vi "Motor Accion.vi"(11 "Tipo Movimiento":string) -> ()   [LabVIEW 2013, in "Proyecto 2 Touch.lvrbt"]
uses:
  Proyecto 2 Touch.lvrbt
  <vilib>/NXT/LegoClasses/BrickReference/BrickReference.lvclass
  <vilib>/NXT/Subs/LVHSConnector.ctl
  <vilib>/NXT/NXTIO Xnodes/NXTIOXNode/NXTIO.xnode
  <vilib>/NXT/NXTIO Xnodes/AddressXNode/NXTIOAddress.xnode
  <vilib>/NXT/Block Support/NXT_OutputPort.ctl
  <vilib>/NXT/NXTIO Xnodes/NXTIONodeSubVIs/NXTMoveMotors.vi
  <vilib>/NXT/NXTIO Xnodes/NXTIONodeSubVIs/LEGOResetMotors.vi
  <vilib>/NXT/NXTIO Xnodes/NXTIONodeSubVIs/LEGOStopAllMotors.vi
  <vilib>/NXT/Dual Mode Library/Waits/Wait_Rotation.vi
  <vilib>/NXT/Dual Mode Library/Waits/Wait_Num(msec).vi
  Global Var.vi
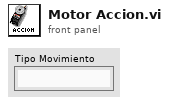
[diagram p1: front panel]
types:
  T1 = typedef "NXT_OutputPort.ctl" = u8
  T2 = typedef "LVHSConnector.ctl" = refnum<class "BrickReference.lvclass">
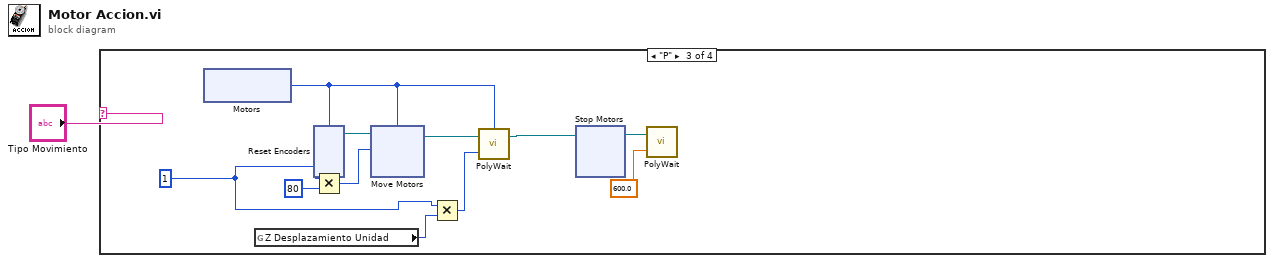
[diagram p0: block diagram]
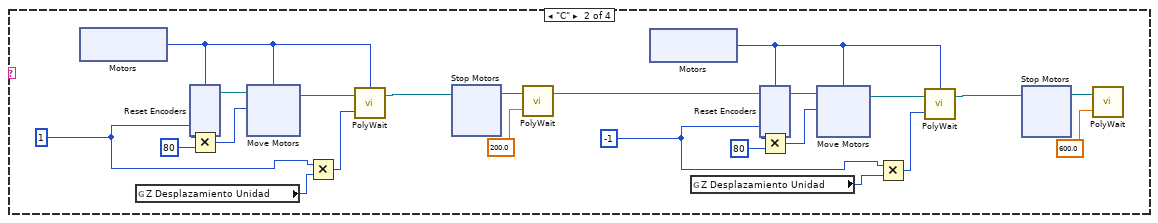
[diagram p3: hidden frame]
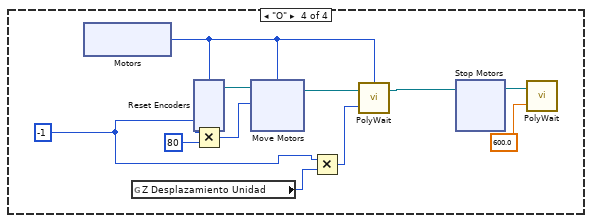
[diagram p4: hidden frame]
diagram:
  n1 = case shown="\"P\"" "Tipo Movimiento" {
    frame Default {
    }
    frame "C" {
      w7 = -1 ("x")
      w17 = 1 ("x")
      n2 = xnode "Motors"() -> ("Motor"=w16:T1)
      n3 = global read "Global Var.vi" "Z Desplazamiento Unidad"() -> (w2:i32)
      n4 = xnode "Reset Encoders"("Motors"=w16) -> ("NXT/EV3"=w23:T2)  [unwired: 1 in]
      n5 = Multiply(x=w17, y=80) -> (x*y=w19:i32)
      n6 = xnode "Move Motors"("Power/Speed 1"=w19, "Motors"=w16, "NXT/EV3"=w23) -> ("NXT/EV3"=w20:T2)
      n7 = Multiply(x=w17, y=w2) -> (x*y=w18:i32)
      n8 = call-poly <vilib>:"PolyWait.vi"("Position Change (180)"=w18, "NXT/EV3"=w20, "Port (Port A)"=w16) -> ("NXT/EV3"=w15:T2)  [unwired: 1 in]
      n9 = xnode "Stop Motors"("NXT/EV3"=w15) -> ("NXT/EV3"=w22:T2)  [unwired: 1 in]
      n10 = call-poly <vilib>:"PolyWait.vi"("Time (100 msec)"=sgl 200.0 ("Time (1 sec)"), "NXT/EV3"=w22) -> ("NXT/EV3"=w4:T2)  [unwired: 2 in]
      n11 = xnode "Motors"() -> ("Motor"=w6:T1)
      n12 = global read "Global Var.vi" "Z Desplazamiento Unidad"() -> (w3:i32)
      n13 = xnode "Reset Encoders"("Motors"=w6, "NXT/EV3"=w4) -> ("NXT/EV3"=w13:T2)
      n14 = Multiply(x=w7, y=80) -> (x*y=w9:i32)
      n15 = xnode "Move Motors"("Power/Speed 1"=w9, "Motors"=w6, "NXT/EV3"=w13) -> ("NXT/EV3"=w10:T2)
      n16 = Multiply(x=w7, y=w3) -> (x*y=w8:i32)
      n17 = call-poly <vilib>:"PolyWait.vi"("Position Change (180)"=w8, "NXT/EV3"=w10, "Port (Port A)"=w6) -> ("NXT/EV3"=w5:T2)  [unwired: 1 in]
      n18 = xnode "Stop Motors"("NXT/EV3"=w5) -> ("NXT/EV3"=w12:T2)  [unwired: 1 in]
      n19 = call-poly <vilib>:"PolyWait.vi"("Time (100 msec)"=sgl 600.0 ("Time (1 sec)"), "NXT/EV3"=w12) -> ()  [unwired: 2 in, 1 out]
    }
    frame "P" {
      w58 = 1 ("x")
      n20 = xnode "Motors"() -> ("Motor"=w57:T1)
      n21 = global read "Global Var.vi" "Z Desplazamiento Unidad"() -> (w55:i32)
      n22 = xnode "Reset Encoders"("Motors"=w57) -> ("NXT/EV3"=w64:T2)  [unwired: 1 in]
      n23 = Multiply(x=w58, y=80) -> (x*y=w60:i32)
      n24 = xnode "Move Motors"("Power/Speed 1"=w60, "Motors"=w57, "NXT/EV3"=w64) -> ("NXT/EV3"=w61:T2)
      n25 = Multiply(x=w58, y=w55) -> (x*y=w59:i32)
      n26 = call-poly <vilib>:"PolyWait.vi"("Position Change (180)"=w59, "NXT/EV3"=w61, "Port (Port A)"=w57) -> ("NXT/EV3"=w56:T2)  [unwired: 1 in]
      n27 = xnode "Stop Motors"("NXT/EV3"=w56) -> ("NXT/EV3"=w63:T2)  [unwired: 1 in]
      n28 = call-poly <vilib>:"PolyWait.vi"("Time (100 msec)"=sgl 600.0 ("Time (1 sec)"), "NXT/EV3"=w63) -> ()  [unwired: 2 in, 1 out]
    }
    frame "O" {
      w84 = -1 ("x")
      n29 = xnode "Motors"() -> ("Motor"=w83:T1)
      n30 = global read "Global Var.vi" "Z Desplazamiento Unidad"() -> (w81:i32)
      n31 = xnode "Reset Encoders"("Motors"=w83) -> ("NXT/EV3"=w90:T2)  [unwired: 1 in]
      n32 = Multiply(x=w84, y=80) -> (x*y=w86:i32)
      n33 = xnode "Move Motors"("Power/Speed 1"=w86, "Motors"=w83, "NXT/EV3"=w90) -> ("NXT/EV3"=w87:T2)
      n34 = Multiply(x=w84, y=w81) -> (x*y=w85:i32)
      n35 = call-poly <vilib>:"PolyWait.vi"("Position Change (180)"=w85, "NXT/EV3"=w87, "Port (Port A)"=w83) -> ("NXT/EV3"=w82:T2)  [unwired: 1 in]
      n36 = xnode "Stop Motors"("NXT/EV3"=w82) -> ("NXT/EV3"=w89:T2)  [unwired: 1 in]
      n37 = call-poly <vilib>:"PolyWait.vi"("Time (100 msec)"=sgl 600.0 ("Time (1 sec)"), "NXT/EV3"=w89) -> ()  [unwired: 2 in, 1 out]
    }
  }
